vi "1. Histogram, Color Space and Threshold.vi"() -> ()   [LabVIEW 2019]
doc: "c 2020 ReMiSYS All rights reserved."
panel:
  in  "offset":i32(slide) scale=0.0..50.0
  in  "Color Mode":enum16{"RGB", "HSL", "HSV", "HSI"}(ring)
  in  "Manual Threshold?":bool
  in  "Blue or Luminance":cluster{i32, i32}(slide)={20, 217} scale=0.0..255.0
  in  "Green or Saturation":cluster{i32, i32}(slide)={20, 233} scale=0.0..255.0
  in  "Red or Hue":cluster{i32, i32}(slide)={42, 99} scale=0.0..255.0
  out "Histogram Graph":u32[][](graph)
  out "Bin Image":T1(plugin-control)
  out "Ori Image":T1(plugin-control)
  in  "Stop (F)":bool
  # "Minimum"
  # "Maximum"
  # "Minimum"
  # "Maximum"
  # "Minimum"
  # "Maximum"
  # "c 2020 ReMiSYS All rights reserved."
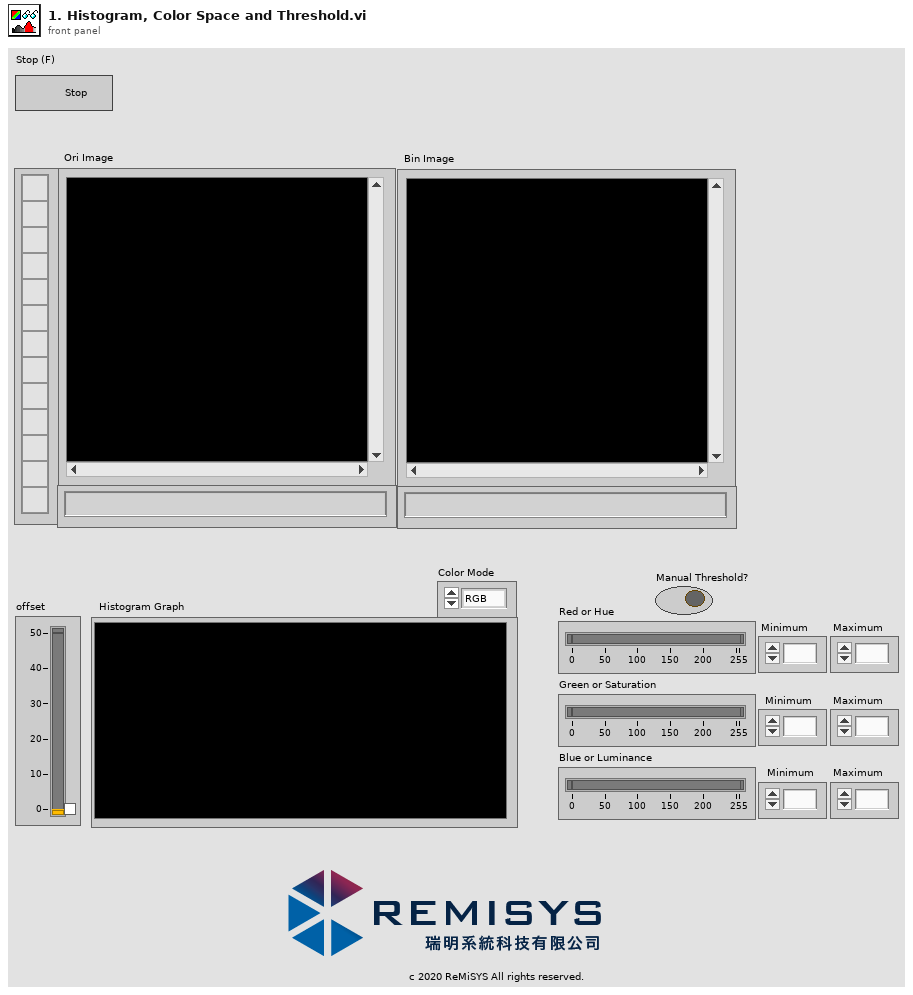
[diagram p1: front panel]
types:
  T1 = typedef "IMAQ Image.ctl" = refnum<image>
  T2 = cluster{"Cluster":cluster{"Numeric Control":i32, "Numeric Control":i32}, "Cluster":cluster{"Numeric Control":i32, "Numeric Control":i32}, "Cluster":cluster{"Numeric Control":i32, "Numeric Control":i32}}
  T3 = cluster{"Numeric Control":i32, "Numeric Control":i32}
  T4 = cluster{"Global Rectangle":i32[], "Contours":cluster{"Contour Type":u32, "ROI Type":u32, "Points":i32[]}[]}
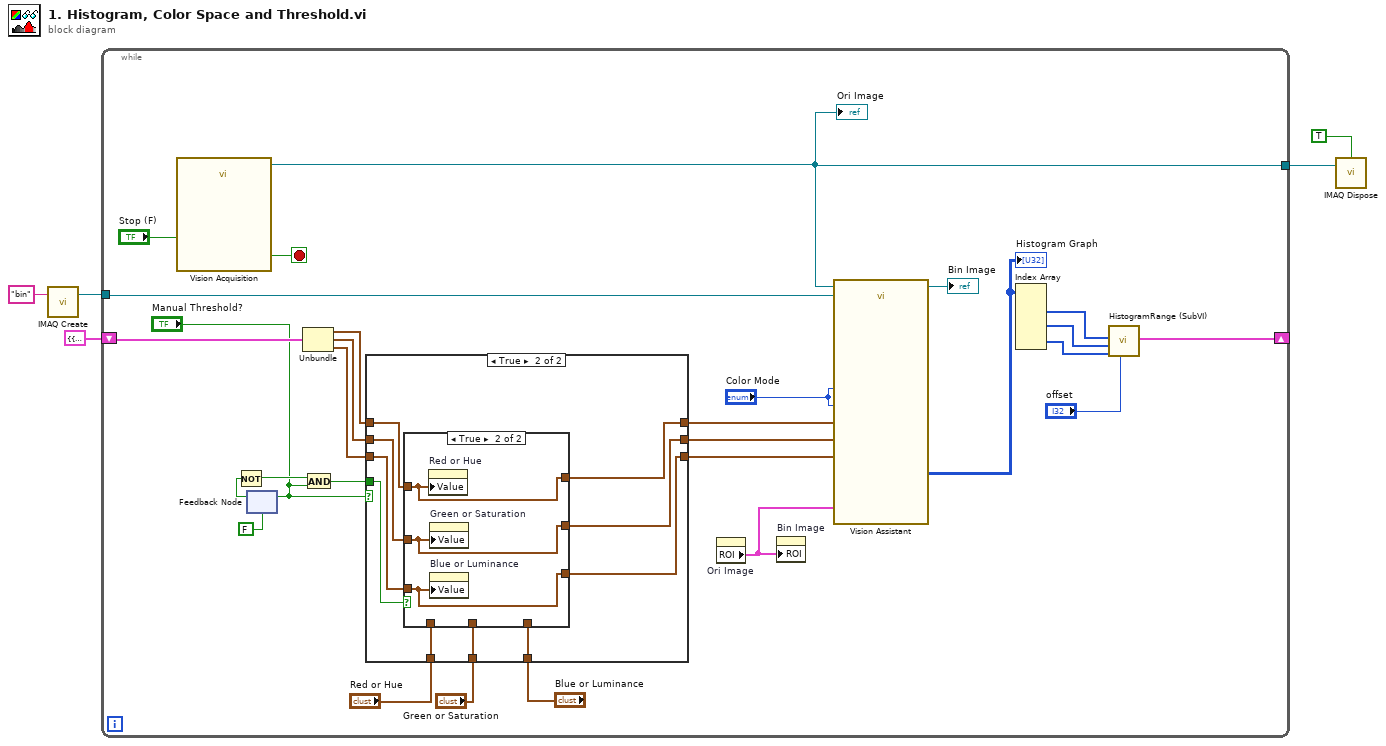
[diagram p0: block diagram]
diagram:
  n1 = call "IMAQ Create"("Image Name"="bin") -> ("New Image"=w3:T1)  [unwired: 4 in, 1 out]
  n2 = while {
    tunnel: [w30] -> w5
    tunnel: w3 -> [w31]
    shift-right: [w12] -> _
    shift-left: T2 {"Cluster"={"Numeric Control"=0, "Numeric Control"=0}, "Cluster"={"Numeric Control"=0, "Numeric Control"=0}, "Cluster"={"Numeric Control"=0, "Numeric Control"=0}} ("Output Range") -> [w13]
    stop <- w32 stop-if-true
    n3 = call "Vision Acquisition"("Stop (F)"="Stop (F)") -> ("Image Out"=w30:T1, "Stopped"=w32:bool)  [unwired: 24 in, 1 out]
    "Ori Image" <- w30
    n4 = feedback #1(FALSE ("Manual Threshold?")) -> (w20:bool)
    n5 = Not(x=w20) -> (.not. x?=w7:bool)
    n6 = feedback-in #1("Manual Threshold?") -> ()
    n7 = Unbundle(w13) -> ("Cluster"=w16:T3, "Cluster"=w15:T3, "Cluster"=w14:T3)
    n8 = And(x=w7, y="Manual Threshold?") -> (x .and. y?=w21:bool)
    n9 = case shown="True" "Manual Threshold?" {
      tunnel: [w36 w46] -> w27
      tunnel: [w35 w45] -> w26
      tunnel: [w34 w44] -> w25
      tunnel: w16 -> [w36 w42]
      tunnel: w15 -> [w35 w40]
      tunnel: w14 -> [w34 w41]
      tunnel: w21 -> [_ w43]
      tunnel: "Blue or Luminance" -> [_ w39]
      tunnel: "Green or Saturation" -> [_ w38]
      tunnel: "Red or Hue" -> [_ w37]
      frame False {
      }
      frame True {
        n10 = case shown="True" w43 {
          tunnel: [w47 w52] -> w46
          tunnel: [w48 w50] -> w45
          tunnel: [w49 w51] -> w44
          tunnel: w42 -> [_ w52]
          tunnel: w41 -> [_ w51]
          tunnel: w40 -> [_ w50]
          tunnel: w39 -> [w49 _]
          tunnel: w38 -> [w48 _]
          tunnel: w37 -> [w47 _]
          frame False {
          }
          frame True {
            n11 = property on="Red or Hue" class="Slide (strict)"("Value"=w52) -> ()  [unwired: 2 in, 2 out]
            n12 = property on="Green or Saturation" class="Slide (strict)"("Value"=w50) -> ()  [unwired: 2 in, 2 out]
            n13 = property on="Blue or Luminance" class="Slide (strict)"("Value"=w51) -> ()  [unwired: 2 in, 2 out]
          }
        }
      }
    }
    n14 = property on="Ori Image" class="ImageControl"() -> ("ROI"=w28:T4)  [unwired: 2 in, 2 out]
    n15 = property on="Bin Image" class="ImageControl"("ROI"=w28) -> ()  [unwired: 2 in, 2 out]
    n16 = call "Vision Assistant"("Image In"=w30, "Image Dst"=w31, "Color Mode (Histogram 1)"="Color Mode", "Color Mode (Color Threshold 1)"="Color Mode", "Red or Hue Range (Color Threshold 1)"=w27, "Green or Sat Range (Color Threshold 1)"=w26, "Blue or Luma or Val or Inten Range (Color Threshold 1)"=w25, "ROI Descriptor (Histogram 1)"=w28) -> ("Image Out"=→"Bin Image":T1, "Histogram (Histogram 1)"=w23:u32[][])  [unwired: 16 in, 2 out]
    "Histogram Graph" <- w23
    n17 = Index Array(array=w23) -> (element #1=w22:u32[], element #2=w18:u32[], element #3=w17:u32[])  [unwired: 6 in]
    n18 = call "HistogramRange (SubVI).vi"("offset"="offset", "Histogram Graph3"=w17, "Histogram Graph2"=w18, "Histogram Graph1"=w22) -> ("Output Range"=w12:T2)  [unwired: 7 in]
  }
  n19 = call "IMAQ Dispose"("All Images? (No)"=TRUE, "Image"=w5) -> ()  [unwired: 4 in, 1 out]
